vi "Update Test Schema.vi"(8 "error in (no error)":errorcluster, 11 "Post Analysis in":refnum<class "Post Analysis.lvclass">) -> (0 "error out":errorcluster, 3 "Post Analysis out":refnum<class "Post Analysis.lvclass">)   [LabVIEW 2023, in "Data Analysis.lvlib" / "Post Analysis.lvlib" / "Post Analysis.lvclass"]
uses:
  Post Analysis.lvclass
  Post Analysis.lvclass/Post Analysis.ctl
  HardwareAbstractionLayer_LVOOP/Database/Database.lvclass
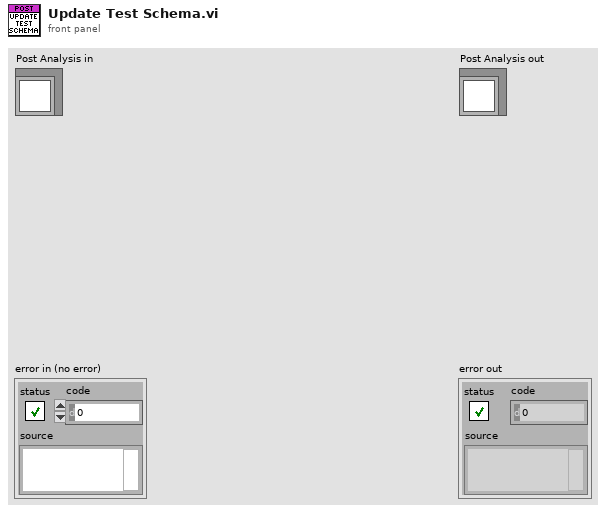
[diagram p1: front panel]
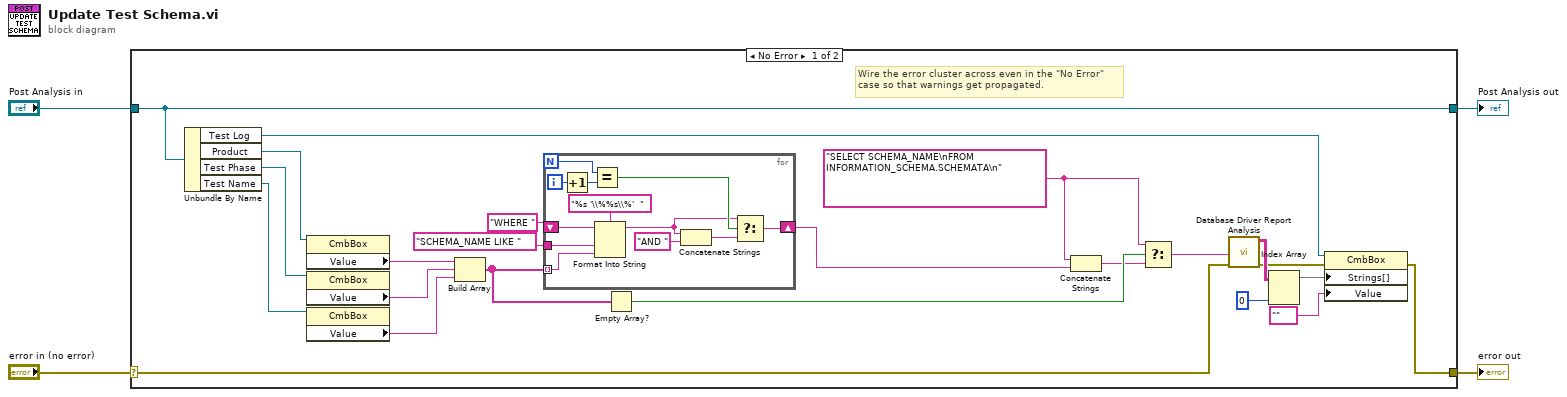
[diagram p0: block diagram]
diagram:
  n1 = case shown="No Error" "error in (no error)" {
    selector: "error in (no error)" -> [w20 w41]
    tunnel: [w19 w41] -> w3
    tunnel: [w22 w40] -> w1
    tunnel: "Post Analysis in" -> [w22 w40]
    frame No Error {
      w11 = "SELECT SCHEMA_NAME\nFROM INFORMATION_SCHEMA.SCHEMATA\n" ("SQL query")
      # "Wire the error cluster across even in the \"No Error\"\ncase so that warnings get propagated."
      n2 = Unbundle By Name(w22) -> ("Test Log"=w21:refnum<vi>, "Product"=w18:refnum<vi>, "Test Phase"=w17:refnum<vi>, "Test Name"=w16:refnum<vi>)
      n3 = property class="CmbBox"(reference=w18) -> ("Value"=w15:string)  [unwired: 1 in, 2 out]
      n4 = property class="CmbBox"(reference=w17) -> ("Value"=w14:string)  [unwired: 1 in, 2 out]
      n5 = property class="CmbBox"(reference=w16) -> ("Value"=w13:string)  [unwired: 1 in, 2 out]
      n6 = Build Array(w15, w14, w13) -> (w7:string[])
      n7 = for {
        N -> [w34]
        tunnel: w7 -> [w36] mode=indexing
        shift-right: [w29] -> w6
        shift-left: "WHERE " -> [w39]
        tunnel: "SCHEMA_NAME LIKE " -> [w37]
        i -> [w35]
        n8 = Increment(x=w35) -> (x+1=w28:i32)
        n9 = Equal?(x=w34, y=w28) -> (x = y?=w32:bool)
        n10 = Format Into String(format string="%s '\\%%s\\%'  ", initial string=w39, w37, w36) -> (resulting string=w31:string)  [unwired: 1 in, 1 out]
        n11 = Concatenate Strings(w31, "AND " ("string")) -> (w30:string)
        n12 = Select(t=w31, s=w32, f=w30) -> (s? t:f=w29:string)
      }
      n13 = Empty Array?(array=w7) -> (empty?=w12:bool)
      n14 = Concatenate Strings(w11, w6) -> (w10:string)
      n15 = Select(t=w11, s=w12, f=w10) -> (s? t:f=w5:string)
      n16 = call "Database Driver Report Analysis.vi"("error in"=w20, "SQL query"=w5) -> ("error out"=w25:errorcluster, "data"=w27:string[][])  [unwired: 6 in, 2 out]
      n17 = Index Array(array=w27, index (col)=0 ("disabled index (col)")) -> (element=w24:string[])  [unwired: 1 in]
      n18 = property class="CmbBox"(reference=w21, error in=w25, "Strings[]"=w24, "Value"="" ("Test Log(Schema)")) -> (error out=w19:errorcluster)  [unwired: 1 out]
    }
    frame Error {
    }
  }
  "error out" <- w3
  "Post Analysis out" <- w1
